vi "getFinalAcquisitionTimings.vi"(8 "error in (no error)":errorcluster, 11 "ICCameraAcquisitor.lvclass in":refnum<class "ICCameraAcquisitor.lvclass">) -> (0 "error out":errorcluster, 2 "Final Acquisition Timings":T1, 3 "ICCameraAcquisitor.lvclass out":refnum<class "ICCameraAcquisitor.lvclass">)   [LabVIEW 2011, in "Hardware.lvlib" / "Channels.lvlib" / "ICCameraAcquisitor.lvclass"]
uses:
  ICCameraAcquisitor.lvclass
  ICCameraAcquisitor.lvclass/ICCameraAcquisitor.ctl
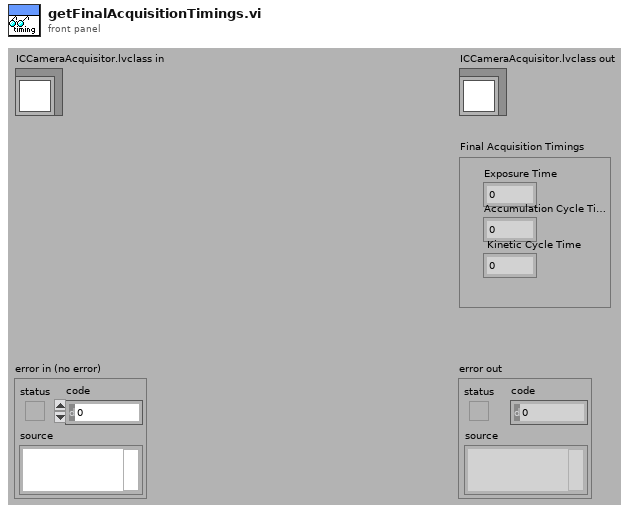
[diagram p1: front panel]
types:
  T1 = cluster{"Exposure Time":dbl, "Accumulation Cycle Time":dbl, " Kinetic Cycle Time":dbl}
  T2 = enum16{"Brightness", "Color Enable", "Contrast", "Exposure", "Focus", "Gain", "Gamma", "Hue", "Iris", "Pan", "Roll", "Saturation", "Sharpness", "Tilt", "Whitebalance", "Zoom", "Whitebalance Blue", "Whitebalance Red"}
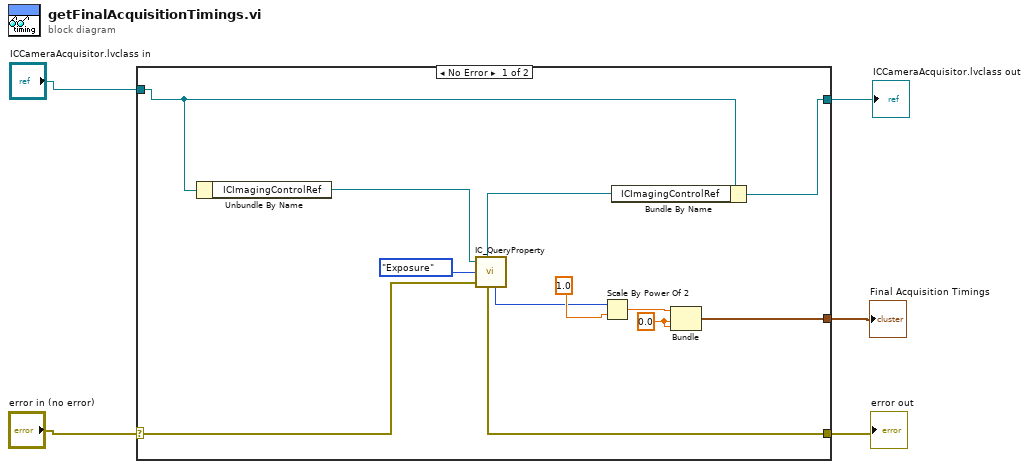
[diagram p0: block diagram]
diagram:
  n1 = case shown="No Error" "error in (no error)" {
    selector: "error in (no error)" -> [w12 w18]
    tunnel: [w11 w18] -> w4
    tunnel: "ICCameraAcquisitor.lvclass in" -> [w15 w19]
    tunnel: [w14 w19] -> w2
    tunnel: [w6 _] -> w1
    frame No Error {
      w7 = 0.0
      n2 = Unbundle By Name(w15) -> ("ICImagingControlRef"=w16:refnum<k7>)
      n3 = call <userlib>:"IC_QueryProperty.vi"("ICImagingControl In"=w16, "Property"=T2."Exposure", "Error In (no error)"=w12) -> ("ICImagingControl Out"=w13:refnum<k7>, "Error Out"=w11:errorcluster, "Value"=w9:i32)  [unwired: 5 out]
      n4 = Scale By Power Of 2(n=w9, x=1.0) -> (x*2^n=w8:dbl)
      n5 = Bundle By Name(cluster=w15, "ICImagingControlRef"=w13) -> (w14:refnum<class "ICCameraAcquisitor.lvclass">)
      n6 = Bundle(w8, w7, w7) -> (w6:cluster{dbl, dbl, dbl})  [unwired: 1 in]
    }
    frame Error {
    }
  }
  "error out" <- w4
  "ICCameraAcquisitor.lvclass out" <- w2
  "Final Acquisition Timings" <- w1
